vi "LDA_header.vi"() -> (0 "LDA Header string":string)   [LabVIEW 2011]
uses:
  Globals/Meas_global.vi
  Globals/LDA_meas_global_1.vi
  Globals/LDA_meas_global_2.vi
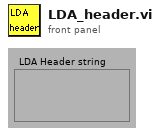
[diagram p1: front panel]
types:
  T1 = typedef "LDA_Setup.ctl" = cluster{"dimensions":enum16{"1D", "2D"}, "Analogue Freq Multiplier":dbl}
  T2 = typedef "BSA_info_Cluster.ctl" = cluster{"GPIB Address":string, "No of Check Bytes":i32, "Extra Info":string, "COLOUR":u32, "Wavelength (nm)":dbl}
  T3 = cluster{"Arrival time clock":enum16{"External", "Internal"}, "Clock source":enum16{"Slave", "Master", "Private"}, "Coincidence":enum16{"Slave", "Master", "Private"}}
  T4 = cluster{"Dead time (s)":dbl, "Duty cycle (%)":dbl, "Data collection mode":enum16{"Burst", "Contiuous", "Dead time", "External"}}
  T5 = enum16{"Burst", "Contiuous", "Dead time", "External"}
  T6 = cluster{"Burst criterion":enum16{"Envelope", "Pedestal", "Env and ped"}, "Oversize reject level":enum16{"1 (disabled)", "2", "3", "4", "5", "6", "7", "8", "9"}, "Pedestal attenuation":enum16{"0", "6", "12", "18"}, "Record length":enum16{"8", "16", "32", "64"}, "Quality factor":i16}
  T7 = enum16{"1 (disabled)", "2", "3", "4", "5", "6", "7", "8", "9"}
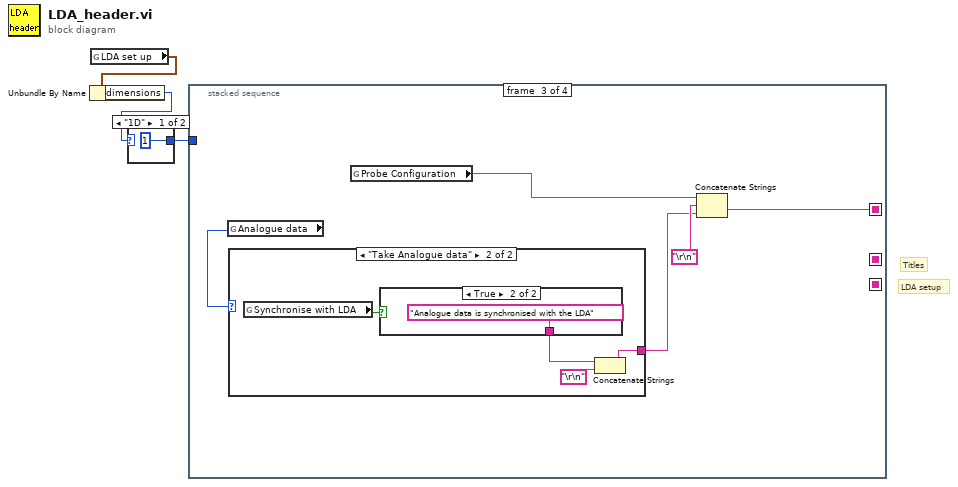
[diagram p0: block diagram]
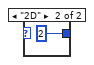
[diagram p2: hidden frame]
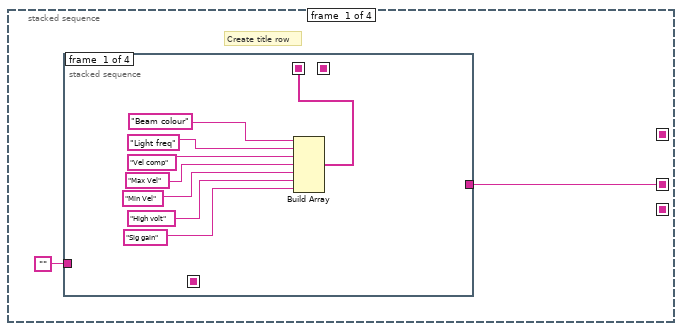
[diagram p3: hidden frame]
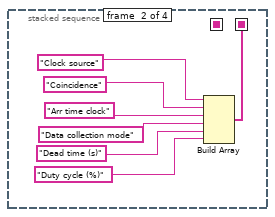
[diagram p4: hidden frame]
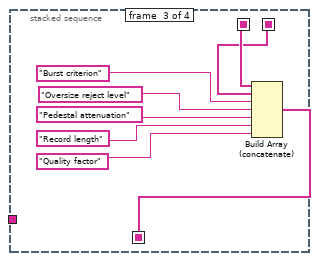
[diagram p5: hidden frame]
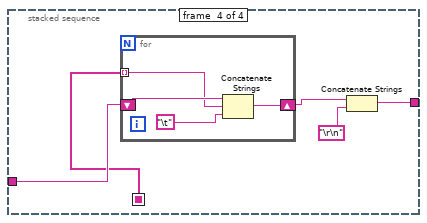
[diagram p6: hidden frame]
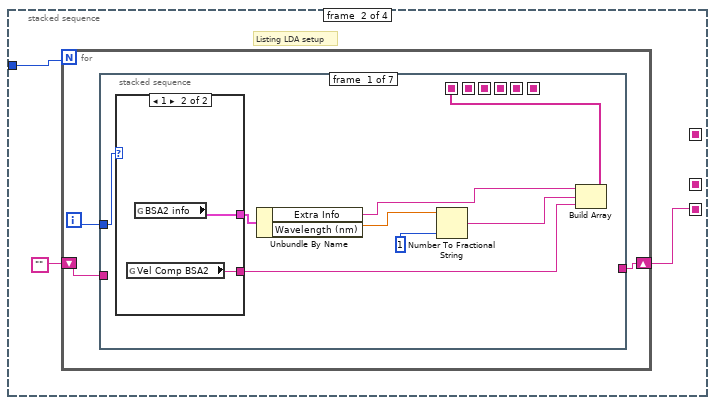
[diagram p7: hidden frame]
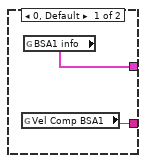
[diagram p8: hidden frame]
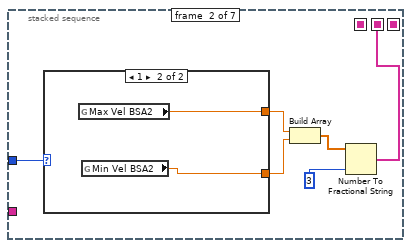
[diagram p9: hidden frame]
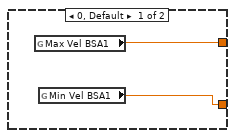
[diagram p10: hidden frame]
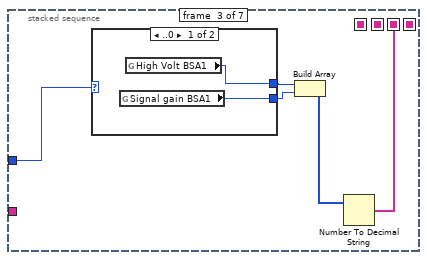
[diagram p11: hidden frame]
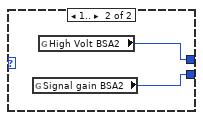
[diagram p12: hidden frame]
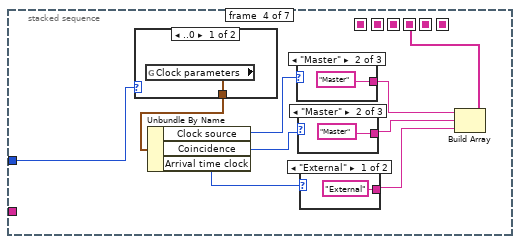
[diagram p13: hidden frame]
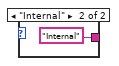
[diagram p14: hidden frame]
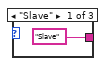
[diagram p15: hidden frame]
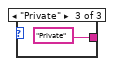
[diagram p16: hidden frame]
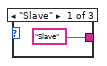
[diagram p17: hidden frame]
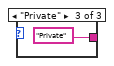
[diagram p18: hidden frame]
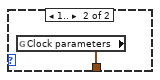
[diagram p19: hidden frame]
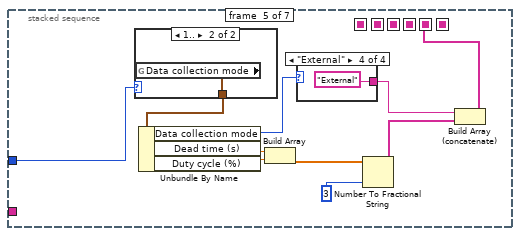
[diagram p20: hidden frame]
diagram:
  # "LDA setup"
  # "Titles"
  n1 = global read "Meas_global.vi" "LDA set up"() -> (w2:T1)
  n2 = Unbundle By Name(w2) -> ("dimensions"=w1:enum16{"1D", "2D"})
  n3 = case shown="\"1D\"" w1 {
    tunnel: [1 2] -> w3
    frame "1D" {
    }
    frame "2D" {
    }
  }
  n4 = stacked-sequence {
    seq-local: [w7 _ _ _] -> [_ _ _ w175]
    seq-local: [_ w42 _ _] -> [_ _ _ w174]
    seq-local: [_ _ w165 _] -> [_ _ _ w177]
    tunnel: w3 -> [_ w40 _ _]
    frame #0 {
      # "Create title row"
      n5 = stacked-sequence {
        seq-local: [w8 _ _ _] -> [_ _ w25 _]
        seq-local: [_ w16 _ _] -> [_ _ w24 _]
        seq-local: [_ _ w23 _] -> [_ _ _ w34]
        tunnel: "" -> [_ _ _ w35]
        tunnel: [_ _ _ w32] -> w7
        frame #0 {
          n6 = Build Array("Beam colour", "Light freq", "Vel comp", "Max Vel", "Min Vel", "High volt", "Sig gain") -> (w8:string[])
        }
        frame #1 {
          n7 = Build Array("Clock source", "Coincidence", "Arr time clock", "Data collection mode", "Dead time (s)", "Duty cycle (%)") -> (w16:string[])
        }
        frame #2 {
          n8 = Build Array (concatenate)(w25, w24, "Burst criterion", "Oversize reject level", "Pedestal attenuation", "Record length", "Quality factor") -> (w23:string[])
        }
        frame #3 {
          n9 = for {
            shift-right: [w38] -> w33
            shift-left: w35 -> [w39]
            tunnel: w34 -> [w36] mode=indexing
            n10 = Concatenate Strings(w39, w36, "\t") -> (w38:string)
          }
          n11 = Concatenate Strings(w33, "\r\n") -> (w32:string)
        }
      }
    }
    frame #1 {
      # "Listing LDA setup"
      n12 = for {
        N: w40 -> [_]
        shift-right: [w43] -> w42
        shift-left: "" -> [w44]
        i -> [w45]
        n13 = stacked-sequence {
          seq-local: [_ w62 _ _ _ _ _] -> [_ _ _ _ _ _ w156]
          seq-local: [w49 _ _ _ _ _ _] -> [_ _ _ _ _ _ w157]
          seq-local: [_ _ w70 _ _ _ _] -> [_ _ _ _ _ _ w155]
          seq-local: [_ _ _ w77 _ _ _] -> [_ _ _ _ _ _ w154]
          seq-local: [_ _ _ _ w96 _ _] -> [_ _ _ _ _ _ w153]
          seq-local: [_ _ _ _ _ w112 _] -> [_ _ _ _ _ _ w152]
          tunnel: w45 -> [w53 w58 w72 w85 w105 w124 _]
          tunnel: w44 -> [_ _ _ _ _ _ w150]
          tunnel: [_ _ _ _ _ _ w149] -> w43
          frame #0 {
            n14 = case shown="1" w53 {
              tunnel: [w55 w57] -> w48
              tunnel: [w54 w56] -> w47
              frame 0, Default {
                n15 = global read "LDA_meas_global_1.vi" "Vel Comp BSA1"() -> (w54:string)
                n16 = global read "LDA_meas_global_1.vi" "BSA1 info"() -> (w55:T2)
              }
              frame 1 {
                n17 = global read "LDA_meas_global_2.vi" "Vel Comp BSA2"() -> (w56:string)
                n18 = global read "LDA_meas_global_2.vi" "BSA2 info"() -> (w57:T2)
              }
            }
            n19 = Unbundle By Name(w48) -> ("Extra Info"=w46:string, "Wavelength (nm)"=w51:dbl)
            n20 = Number To Fractional String(number=w51, precision (6)=1) -> (F-format string=w50:string)  [unwired: 2 out]
            n21 = Build Array(w46, w50, w47) -> (w49:string[])
          }
          frame #1 {
            n22 = case shown="1" w58 {
              tunnel: [w65 w67] -> w61
              tunnel: [w64 w66] -> w60
              frame 0, Default {
                n23 = global read "LDA_meas_global_1.vi" "Max Vel BSA1"() -> (w65:dbl)
                n24 = global read "LDA_meas_global_1.vi" "Min Vel BSA1"() -> (w64:dbl)
              }
              frame 1 {
                n25 = global read "LDA_meas_global_2.vi" "Max Vel BSA2"() -> (w67:dbl)
                n26 = global read "LDA_meas_global_2.vi" "Min Vel BSA2"() -> (w66:dbl)
              }
            }
            n27 = Build Array(w61, w60) -> (w59:dbl[])
            n28 = Number To Fractional String(number=w59, precision (6)=3) -> (F-format string=w62:string[])  [unwired: 2 out]
          }
          frame #2 {
            n29 = case shown="..0" w72 {
              tunnel: [w74 w76] -> w69
              tunnel: [w73 w75] -> w68
              frame ..0 {
                n30 = global read "LDA_meas_global_1.vi" "Signal gain BSA1"() -> (w73:i16)
                n31 = global read "LDA_meas_global_1.vi" "High Volt BSA1"() -> (w74:i16)
              }
              frame 1.. {
                n32 = global read "LDA_meas_global_2.vi" "Signal gain BSA2"() -> (w75:i16)
                n33 = global read "LDA_meas_global_2.vi" "High Volt BSA2"() -> (w76:i16)
              }
            }
            n34 = Build Array(w69, w68) -> (w71:i16[])
            n35 = Number To Decimal String(number=w71) -> (decimal integer string=w70:string[])  [unwired: 1 out]
          }
          frame #3 {
            n36 = case shown="..0" w85 {
              tunnel: [w94 w95] -> w84
              frame ..0 {
                n37 = global read "LDA_meas_global_1.vi" "Clock parameters"() -> (w94:T3)
              }
              frame 1.. {
                n38 = global read "LDA_meas_global_2.vi" "Clock parameters"() -> (w95:T3)
              }
            }
            n39 = Unbundle By Name(w84) -> ("Clock source"=w82:enum16{"Slave", "Master", "Private"}, "Coincidence"=w83:enum16{"Slave", "Master", "Private"}, "Arrival time clock"=w79:enum16{"External", "Internal"})
            n40 = case shown="\"Master\"" w82 {
              tunnel: ["Slave" "Master" "Private"] -> w81
              frame "Slave" {
              }
              frame "Master" {
              }
              frame "Private" {
              }
            }
            n41 = case shown="\"Master\"" w83 {
              tunnel: ["Slave" "Master" "Private"] -> w80
              frame "Slave" {
              }
              frame "Master" {
              }
              frame "Private" {
              }
            }
            n42 = case shown="\"External\"" w79 {
              tunnel: ["External" "Internal"] -> w78
              frame "External" {
              }
              frame "Internal" {
              }
            }
            n43 = Build Array(w81, w80, w78) -> (w77:string[])
          }
          frame #4 {
            n44 = case shown="1.." w105 {
              tunnel: [w110 w111] -> w104
              frame ..0 {
                n45 = global read "LDA_meas_global_1.vi" "Data collection mode"() -> (w110:T4)
              }
              frame 1.. {
                n46 = global read "LDA_meas_global_2.vi" "Data collection mode"() -> (w111:T4)
              }
            }
            n47 = Unbundle By Name(w104) -> ("Data collection mode"=w103:T5, "Dead time (s)"=w99:dbl, "Duty cycle (%)"=w98:dbl)
            n48 = Build Array(w99, w98) -> (w100:dbl[])
            n49 = case shown="\"External\"" w103 {
              tunnel: ["Burst" "Continuous" "Dead time" "External"] -> w102
              frame "Burst" {
              }
              frame "Contiuous" {
              }
              frame "Dead time" {
              }
              frame "External" {
              }
            }
            n50 = Number To Fractional String(number=w100, precision (6)=3) -> (F-format string=w97:string[])  [unwired: 2 out]
            n51 = Build Array (concatenate)(w102, w97) -> (w96:string[])
          }
          frame #5 {
            n52 = case shown="1.." w124 {
              tunnel: [w145 w146] -> w123
              frame ..0 {
                n53 = global read "LDA_meas_global_1.vi" "Analysis parameters"() -> (w145:T6)
              }
              frame 1.. {
                n54 = global read "LDA_meas_global_2.vi" "Analysis parameters"() -> (w146:T6)
              }
            }
            n55 = Unbundle By Name(w123) -> ("Burst criterion"=w121:enum16{"Envelope", "Pedestal", "Env and ped"}, "Oversize reject level"=w122:T7, "Pedestal attenuation"=w118:enum16{"0", "6", "12", "18"}, "Record length"=w116:enum16{"8", "16", "32", "64"}, "Quality factor"=w115:i16)
            n56 = case shown="\"Envelope\"" w121 {
              tunnel: ["Envelope" "Pedestal" "Env and ped"] -> w120
              frame "Envelope" {
              }
              frame "Pedestal" {
              }
              frame "Env and ped" {
              }
            }
            n57 = case shown="\"1 (disabled)\"" w122 {
              tunnel: ["1 (disabled)" "2" "3" "4" "5" "6" "7" "8" "9"] -> w119
              frame "1 (disabled)" {
              }
              frame "2" {
              }
              frame "3" {
              }
              frame "4" {
              }
              frame "5" {
              }
              frame "6" {
              }
              frame "7" {
              }
              frame "8" {
              }
              frame "9" {
              }
            }
            n58 = case shown="\"0\"" w118 {
              tunnel: ["0" "6" "12" "18"] -> w117
              frame "0" {
              }
              frame "6" {
              }
              frame "12" {
              }
              frame "18" {
              }
            }
            n59 = Number To Decimal String(number=w115) -> (decimal integer string=w114:string)  [unwired: 1 out]
            n60 = case shown="\"64\"" w116 {
              tunnel: ["8" "16" "32" "64"] -> w113
              frame "8" {
              }
              frame "16" {
              }
              frame "32" {
              }
              frame "64" {
              }
            }
            n61 = Build Array(w120, w119, w117, w113, w114) -> (w112:string[])
          }
          frame #6 {
            n62 = Build Array (concatenate)(w157, w156, w155, w154, w153, w152) -> (w151:string[])
            n63 = for {
              shift-right: [w160] -> w147
              shift-left: w150 -> [w161]
              tunnel: w151 -> [w158] mode=indexing
              n64 = Concatenate Strings(w161, w158, "\t") -> (w160:string)
            }
            n65 = Concatenate Strings(w147, "\r\n") -> (w149:string)
          }
        }
      }
    }
    frame #2 {
      n66 = global read "Meas_global.vi" "Analogue data"() -> (w166:enum16{"No Analogue data", "Take Analogue data"})
      n67 = case shown="\"Take Analogue data\"" w166 {
        tunnel: ["" w170] -> w163
        frame "No Analogue data" {
        }
        frame "Take Analogue data" {
          n68 = global read "Meas_global.vi" "Synchronise with LDA"() -> (w171:bool)
          n69 = case shown="True" w171 {
            tunnel: ["Analogue data is not synchronised with the LDA" "Analogue data is synchronised with the LDA"] -> w169
            frame False {
            }
            frame True {
            }
          }
          n70 = Concatenate Strings(w169, "\r\n") -> (w170:string)
        }
      }
      n71 = global read "LDA_meas_global_1.vi" "Probe Configuration"() -> (w162:string)
      n72 = Concatenate Strings(w162, "\r\n", w163) -> (w165:string)
    }
    frame #3 {
      n73 = Concatenate Strings(w177, w175, w174) -> (→"LDA Header string":string)
    }
  }
